vi "ReconcileAlarmUpdate.vi"(8 "error in (no error)":errorcluster, 10 "Updates":T1[](array[typedef]), 11 "config in":T3) -> (0 "error out":errorcluster, 3 "config out":T3)   [LabVIEW 2017, in "TrendAlarm.lvlib"]
uses:
  <vilib>/addons/InsightCM/Devices/Shared/Common/TrendAlarm/TrendAlarm.lvlib
  <vilib>/addons/InsightCM/Devices/Shared/Common/TrendAlarm/controls/config.ctl
  <vilib>/addons/InsightCM/MessageBus/Base/controls/DeviceTrendAlarmUpdate.ctl
  <vilib>/addons/InsightCM/MessageBus/Base/controls/TrendAlarmTransition.ctl
  <vilib>/addons/InsightCM/Devices/Shared/Common/TrendAlarm/controls/TransitionCache.ctl
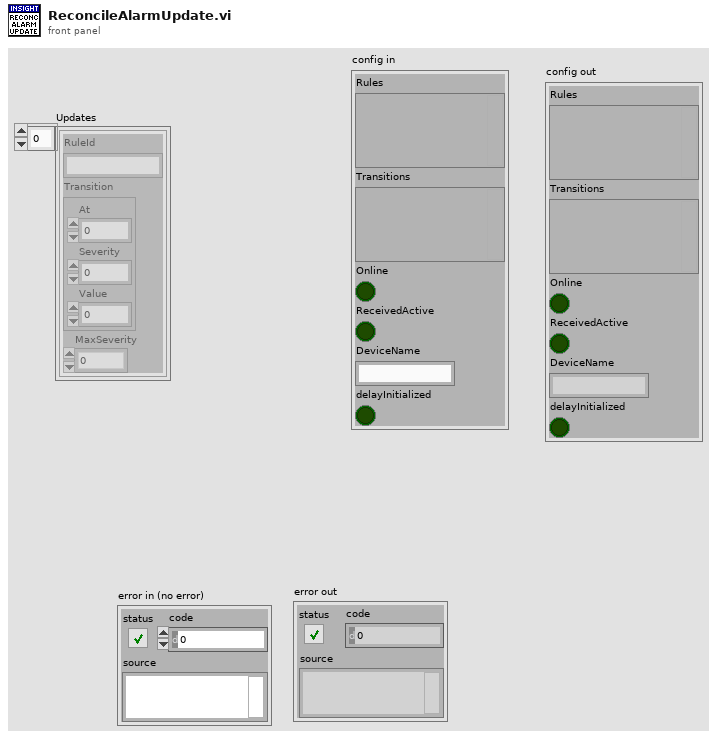
[diagram p1: front panel]
types:
  T1 = typedef "DeviceTrendAlarmUpdate.ctl" = cluster{"RuleId":string, "Transition":T2, "MaxSeverity":i32}
  T2 = typedef "TrendAlarmTransition.ctl" = cluster{"At":i64, "Severity":i32, "Value":dbl}
  T3 = typedef "TrendAlarm.lvlib/config.ctl" = cluster{"Rules":variant, "Transitions":variant, "Online":bool, "ReceivedActive":bool, "DeviceName":string, "delayInitialized":bool}
  T4 = typedef "TrendAlarm.lvlib/TransitionCache.ctl" = cluster{"RuleId":string, "MaxSeverity":i32, "LastTransition":T2, "OnTime":timestamp, "OffTime":timestamp}
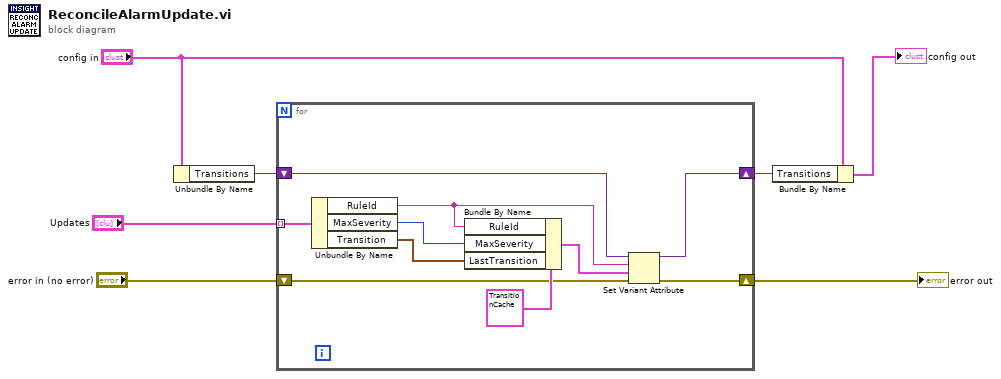
[diagram p0: block diagram]
diagram:
  n1 = Unbundle By Name("config in") -> ("Transitions"=w6:variant)
  n2 = for {
    tunnel: "Updates" -> [w17] mode=indexing
    shift-right: [w14] -> w3
    shift-left: w6 -> [w15]
    shift-right: [w16] -> w5
    shift-left: "error in (no error)" -> [w8]
    n3 = Unbundle By Name(w17) -> ("RuleId"=w13:string, "MaxSeverity"=w11:i32, "Transition"=w12:T2)
    n4 = Bundle By Name(cluster=T4 {"RuleId"="", "MaxSeverity"=0, "LastTransition"={"At"=0, "Severity"=0, "Value"=0.0}, "OnTime"=timestamp(0 s since 1904-01-01), "OffTime"=timestamp(0 s since 1904-01-01)} ("TransitionCache"), "RuleId"=w13, "MaxSeverity"=w11, "LastTransition"=w12) -> (w10:T4)
    n5 = Set Variant Attribute(Variant=w15, name=w13, value=w10, error in=w8) -> (Variant out=w14:variant, error out=w16:errorcluster)  [unwired: 1 out]
  }
  "error out" <- w5
  n6 = Bundle By Name(cluster="config in", "Transitions"=w3) -> (→"config out":T3)
